vi "Configure Baseband Frequency Offset.vi"(8 "error in (no error)":errorcluster, 9 "Baseband Frequency Offset (0 Hz)":dbl, 10 "Modulation Format (1: Dual Modulation)":u16(ring)=1 items=["Dual Modulation"=1, "Dual ARB"=2, "Multitone"=3, "Two-tone"=6], 11 "VISA resource name":refnum<visa-resource-name>) -> (0 "error out":errorcluster, 3 "VISA resource name out":refnum<visa-resource-name>)   [LabVIEW 2011, in "Agilent PSG MXG Series.lvlib"]
doc: "Configures baseband frequency offset.\n\n<B>Notes:</B>\n(1) This VI is valid only in N5182A that installs <B>Option 651</B> or <B>Option 652</B> or <B>Option 654</B> (Internal baseband generator)."
uses:
  Agilent PSG MXG Series.lvlib
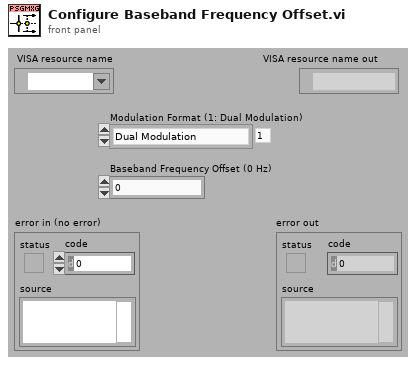
[diagram p1: front panel]
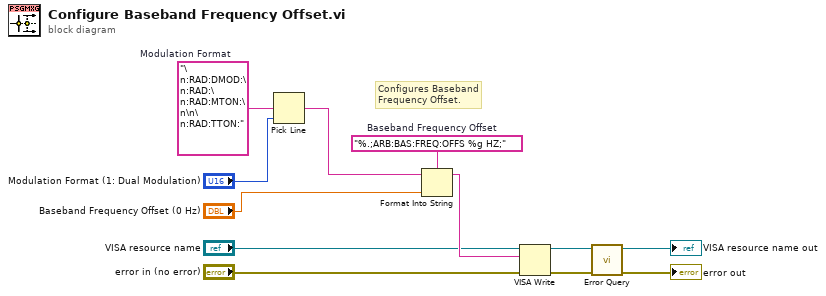
[diagram p0: block diagram]
diagram:
  w10 = "%.;ARB:BAS:FREQ:OFFS %g HZ;"  # Baseband Frequency Offset
  w12 = "\n:RAD:DMOD:\n:RAD:\n:RAD:MTON:\n\n\n:RAD:TTON:"  # Modulation Format
  # "Configures Baseband\nFrequency Offset."
  n1 = Pick Line(multi-line string=w12, line index="Modulation Format (1: Dual Modulation)") -> (output string=w9:string)  [unwired: 1 in]
  n2 = Format Into String(format string=w10, initial string=w9, "Baseband Frequency Offset (0 Hz)") -> (resulting string=w7:string)  [unwired: 1 in, 1 out]
  n3 = VISA Write(VISA resource name="VISA resource name", write buffer=w7, error in (no error)="error in (no error)") -> (VISA resource name out=w6:refnum<visa-resource-name>, error out=w5:errorcluster)  [unwired: 1 out]
  n4 = call "Error Query.vi"("error in (no error)"=w5, "VISA resource name"=w6) -> ("error out"=→"error out":errorcluster, "VISA resource name out"=→"VISA resource name out":refnum<visa-resource-name>)  [unwired: 6 in, 2 out]
